vi "tampon.vi"() -> ()   [LabVIEW 2015]
uses:
  <vilib>/LVH/AR Drone Toolkit/AR Drone.lvlib
  <vilib>/LVH/AR Drone Toolkit/Decode NavData/Typedefs/NavData Demo.ctl
panel:
  out "Battery Remaining":dbl(slide) scale=0.0..100.0
  out "NavData Out":T1
  in  "stop":bool
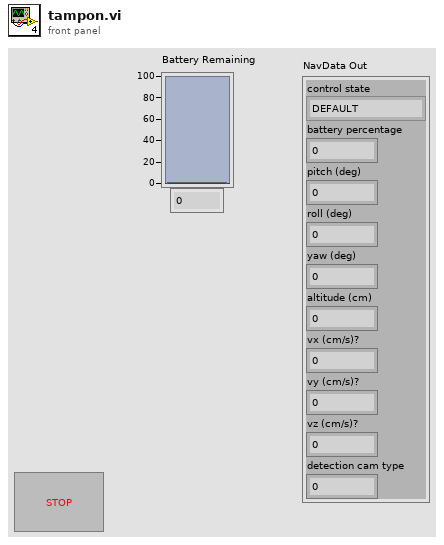
[diagram p1: front panel]
types:
  T1 = typedef "AR Drone.lvlib/NavData Demo.ctl" = cluster{"control state":enum32{"DEFAULT", "INIT", "LANDING", "FLYING", "HOVERING", "TEST", "TRANS_TAKEOFF", "TRANS_GOTOFIX", "TRANS_LANDING"}, "battery percentage":u32, "pitch (deg)":sgl, "roll (deg)":sgl, "yaw (deg)":sgl, "altitude (cm)":u32, "vx (cm/s)?":sgl, "vy (cm/s)?":sgl, "vz (cm/s)?":sgl, "detection cam type":u32}
  T2 = typedef "AR Drone.lvlib/AR Drone Resource.ctl" = cluster{"UDP Control Connection":refnum<k16>, "UDP NavData Connection":refnum<k16>, "UDP Video Connection (Drone 1.0)":refnum<k16>, "TCP Video Connection (Drone 2.0)":refnum<k5>, "TCP Control Port Connection":refnum<k5>, "Drone IP address":string, "Drone Command Port":u16, "Drone NavData Port":u16, "Drone Vid Stream Port":u16, "Drone TCP Control Port":u16, "Home IP address":string, "Home Command Port":u16, "Home NavData Port":u16, "Home Vid Stream Port":u16, "Drone Version":i32, "Drone Index":i32, "Command Sequence":i32}
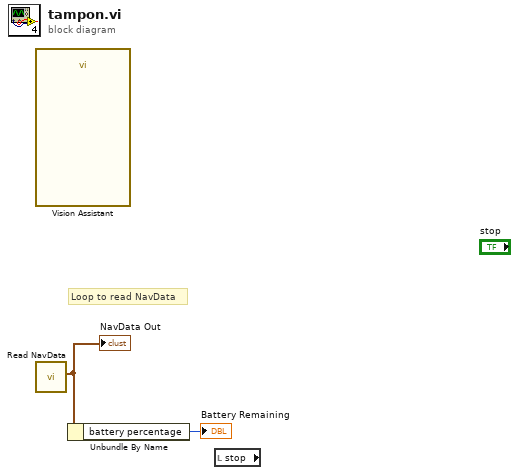
[diagram p0: block diagram]
diagram:
  # "Loop to read NavData"
  n1 = call "Vision Assistant"() -> ()  [unwired: 23 in, 5 out]
  n2 = call <vilib>:"Read NavData.vi"() -> ("error out"=w3:errorcluster, "NavData Out"=w2:T1, "AR Drone Resource Out"=w5:T2, "error in (no error)"=w4:errorcluster, "AR Drone Resource"=w6:T2)  [unwired: 7 in]
  "NavData Out" <- w2
  n3 = Unbundle By Name(w2) -> ("battery percentage"=→"Battery Remaining":u32)
  n4 = local read "stop"() -> ()  [unwired: 1 out]
